vi "Next Rune As UTF-8 Substring.vi"(8 "error in (no error)":errorcluster, 11 "UTF8 in":refnum<class "UTF-8 String.lvclass">) -> (0 "error out":errorcluster, 2 "Rune":string, 3 "UTF8 out":refnum<class "UTF-8 String.lvclass">)   [LabVIEW 2019, in "JKI Unicode.lvlib" / "UTF-8 String.lvclass"]
doc: "JKI Unicode 1.0.0.7\nTomi Maila - JKI\nCopyright (c) 2016, JKI"
uses:
  UTF-8 String.lvclass
  UTF-8 String.lvclass/UTF-8 String.ctl
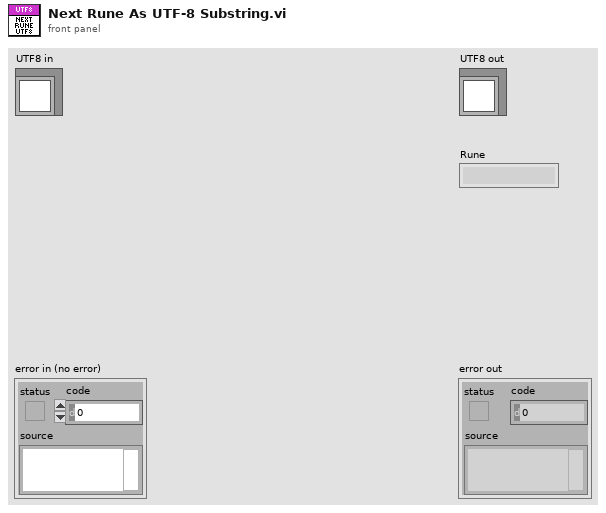
[diagram p1: front panel]
types:
  T1 = typedef "JKI Unicode.lvlib/UTF-8 String.lvclass/Byte Stream.ctl" = u8[]
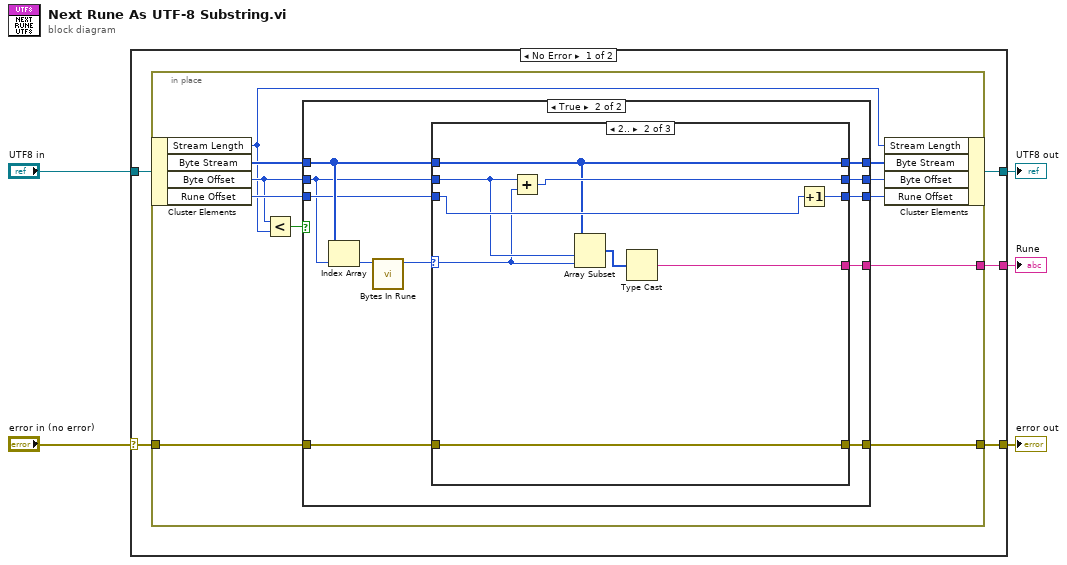
[diagram p0: block diagram]
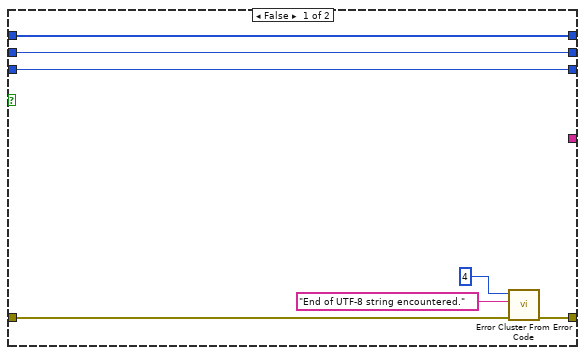
[diagram p2: hidden frame]
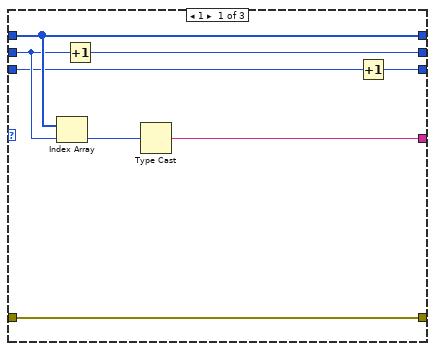
[diagram p3: hidden frame]
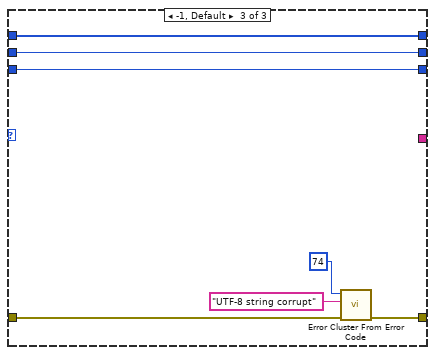
[diagram p4: hidden frame]
diagram:
  n1 = case shown="No Error" "error in (no error)" {
    selector: "error in (no error)" -> [w8 w65]
    tunnel: [w6 w65] -> w4
    tunnel: [w9 w64] -> w2
    tunnel: "UTF8 in" -> [w10 w64]
    tunnel: [w7 _] -> w1
    frame No Error {
      n2 = in-place {
        in-place-border: w8 -> [w16]
        in-place-border: [w18] -> w7
        in-place-border: [w15] -> w6
        n3 = in-place-cluster #1(w10) -> ("Stream Length"=w12:i32, "Byte Stream"=w21:T1, "Byte Offset"=w13:i32, "Rune Offset"=w17:i32)
        n4 = Less?(x=w13, y=w12) -> (x < y?=w11:bool)
        n5 = case shown="True" w11 {
          tunnel: w21 -> [w28 w37]
          tunnel: [w28 w36] -> w20
          tunnel: [w27 w35] -> w19
          tunnel: [_ w34] -> w18
          tunnel: w17 -> [w26 w33]
          tunnel: w16 -> [w24 w32]
          tunnel: [w25 w31] -> w15
          tunnel: [w26 w30] -> w14
          tunnel: w13 -> [w27 w29]
          frame False {
            n6 = call <vilib>:"Error Cluster From Error Code.vi"("error in (no error)"=w24, "error message (\"\")"="End of UTF-8 string encountered." ("error message (\"\")"), "error code (0)"=4) -> ("error out"=w25:errorcluster)  [unwired: 6 in]
          }
          frame True {
            n7 = Index Array(array=w37, index=w29) -> (element=w39:u8)
            n8 = call "Bytes In Rune.vi"("Byte"=w39) -> ("Bytes in Rune"=w38:i8)  [unwired: 10 in]
            n9 = case shown="2.." w38 {
              selector: w38 -> [_ w50 _]
              tunnel: w37 -> [w47 w52 w63]
              tunnel: [w47 w52 w63] -> w36
              tunnel: w29 -> [w46 w51 w62]
              tunnel: [w40 w48 _] -> w34
              tunnel: [w45 w56 w62] -> w35
              tunnel: w33 -> [w42 w53 w57]
              tunnel: w32 -> [w44 w55 w61]
              tunnel: [w44 w55 w60] -> w31
              tunnel: [w43 w54 w57] -> w30
              frame 1 {
                n10 = Index Array(array=w47, index=w46) -> (element=w41:u8)
                n11 = Increment(x=w46) -> (x+1=w45:i32)
                n12 = Type Cast(x=w41) -> (*(type *) &x=w40:string)  [unwired: 1 in]
                n13 = Increment(x=w42) -> (x+1=w43:i32)
              }
              frame 2.. {
                n14 = Add(x=w51, y=w50) -> (x+y=w56:i32)
                n15 = Array Subset(array=w52, index=w51, length=w50) -> (w49:T1)
                n16 = Type Cast(x=w49) -> (*(type *) &x=w48:string)  [unwired: 1 in]
                n17 = Increment(x=w53) -> (x+1=w54:i32)
              }
              frame -1, Default {
                n18 = call <vilib>:"Error Cluster From Error Code.vi"("error in (no error)"=w61, "error message (\"\")"="UTF-8 string corrupt" ("error message (\"\")"), "error code (0)"=74) -> ("error out"=w60:errorcluster)  [unwired: 6 in]
              }
            }
          }
        }
        n19 = in-place-cluster #1("Stream Length"=w12, "Byte Stream"=w20, "Byte Offset"=w19, "Rune Offset"=w14) -> (w9:refnum<class "UTF-8 String.lvclass">)
      }
    }
    frame Error {
    }
  }
  "error out" <- w4
  "UTF8 out" <- w2
  "Rune" <- w1
